vi "Temp Warn SubVI.vi"(8 "error in (no error)":errorcluster, 9 "Min Temperature":dbl, 10 "Max Temperature":dbl, 11 "Current Temperature":dbl) -> (0 "error out":errorcluster, 2 "Boolean":bool, 3 "f":string)   [LabVIEW 2020]
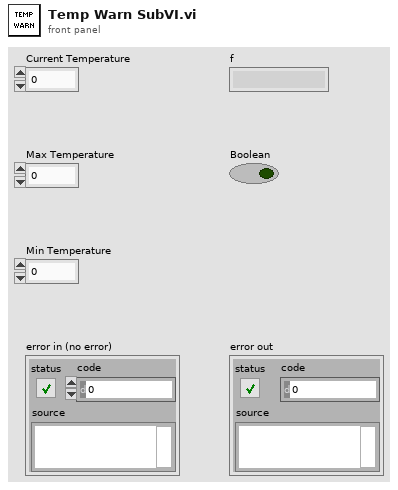
[diagram p1: front panel]
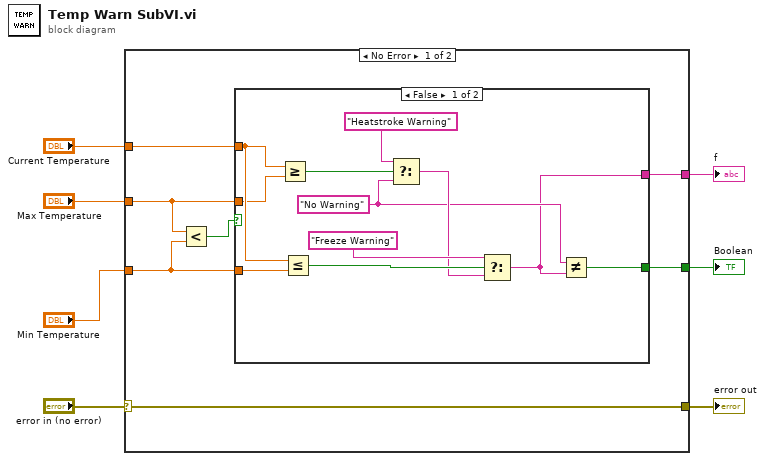
[diagram p0: block diagram]
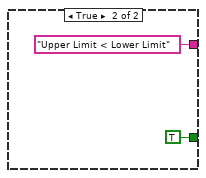
[diagram p2: hidden frame]
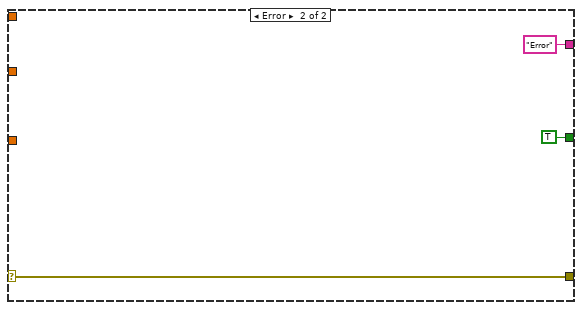
[diagram p3: hidden frame]
diagram:
  n1 = case shown="No Error" "error in (no error)" {
    selector: "error in (no error)" -> [w11 w30]
    tunnel: "Current Temperature" -> [w14 _]
    tunnel: [w13 TRUE] -> w2
    tunnel: "Min Temperature" -> [w8 _]
    tunnel: "Max Temperature" -> [w9 _]
    tunnel: [w12 "Error" ("f")] -> w5
    tunnel: [w11 w30] -> w7
    frame No Error {
      n2 = Less?(x=w9, y=w8) -> (x < y?=w10:bool)
      n3 = case shown="False" w10 {
        tunnel: w14 -> [w24 _]
        tunnel: [w20 TRUE] -> w13
        tunnel: w8 -> [w17 _]
        tunnel: w9 -> [w16 _]
        tunnel: [w15 "Upper Limit < Lower Limit" ("f")] -> w12
        frame False {
          w18 = "No Warning" ("f")
          n4 = Greater Or Equal?(x=w24, y=w16) -> (x >= y?=w25:bool)
          n5 = Less Or Equal?(x=w24, y=w17) -> (x <= y?=w22:bool)
          n6 = Select(t="Heatstroke Warning", s=w25, f=w18) -> (s? t:f=w19:string)
          n7 = Select(t="Freeze Warning", s=w22, f=w19) -> (s? t:f=w15:string)
          n8 = Not Equal?(x=w18, y=w15) -> (x != y?=w20:bool)
        }
        frame True {
        }
      }
    }
    frame Error {
    }
  }
  "error out" <- w7
  "f" <- w5
  "Boolean" <- w2
